vi "~file process.vi"() -> ()   [LabVIEW 2017] (continued)
  "index of next sweep record" <- w5
  "sweep record numbers" <- w1
